vi "IPS Examine Status.vi"(3 "Error In":errorcluster={"status"=FALSE, "code"=1073676294, "source"="VISA Read in Prologix USB GPIB Command.vi"}, 5 "VISA resource name 2":refnum<visa-resource-name>="COM3") -> (0 "Error Out":errorcluster={"status"=FALSE, "code"=1073676294, "source"="VISA Read in Prologix_GPIB_Sample.vi"}, 1 "VISA resource name":refnum<visa-resource-name>="GPIB1::25::INSTR", 2 "Return String from Device (Not all commands return a String)":string="C\r")   [LabVIEW 2013]
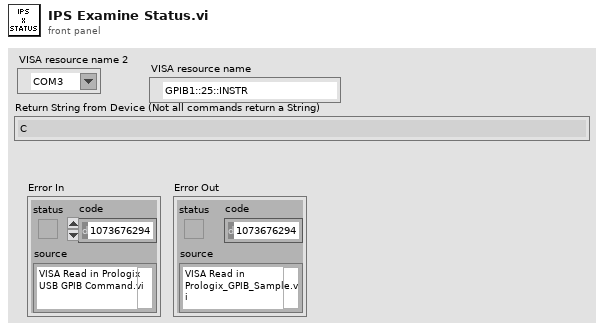
[diagram p1: front panel]
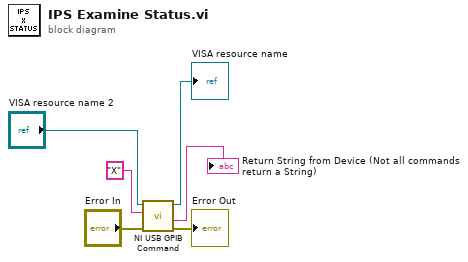
[diagram p0: block diagram]
diagram:
  n1 = call "NI USB GPIB Command.vi"("Error In"="Error In", "String to Send"="X", "VISA resource name"="VISA resource name 2") -> ("Error Out"=→"Error Out":errorcluster, "Return String from Device (Not all commands return a String)"=→"Return String from Device (Not all commands return a String)":string, "VISA resource name"=→"VISA resource name":refnum<visa-resource-name>)  [unwired: 1 in, 1 out]
